vi "create1.vi"(9 "center":i32, 10 "X size":i32, 11 "max Y size":i32) -> (1 "size":i32, 3 "Array":i32[][](array[numeric]))   [LabVIEW 2011]
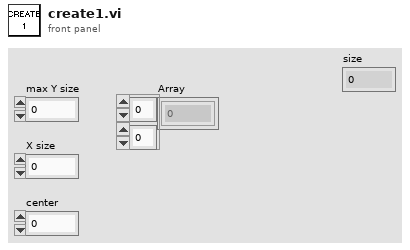
[diagram p1: front panel]
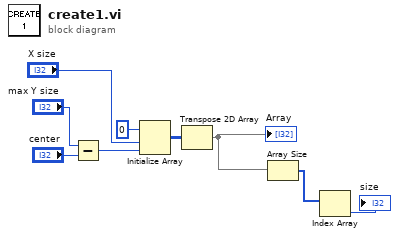
[diagram p0: block diagram]
diagram:
  n1 = Subtract(x="max Y size", y="center") -> (x-y=w4:i32)
  n2 = Initialize Array(0, "X size", w4) -> (w7:i32[][])
  n3 = Transpose 2D Array(2D array=w7) -> (transposed array=w3:i32[][])
  "Array" <- w3
  n4 = Array Size(array=w3) -> (size(s)=w2:i32[])
  n5 = Index Array(array=w2) -> (element=→"size":i32)  [unwired: 1 in]
